vi "Detach Node.vi"(6 "Delete Children?(True)":bool=TRUE, 8 "error in (no error)":errorcluster, 9 "Delete Activate Node(False)":bool, 10 "Node Name":string, 11 "TREE in":refnum<class "MyTreeAPI.lvclass">) -> (0 "error out":errorcluster, 3 "TREE out":refnum<class "MyTreeAPI.lvclass">)   [LabVIEW 2015, in "MyTreeAPI.lvclass"]
uses:
  MyTreeAPI.lvclass
  MyTreeAPI.lvclass/MyTreeAPI.ctl
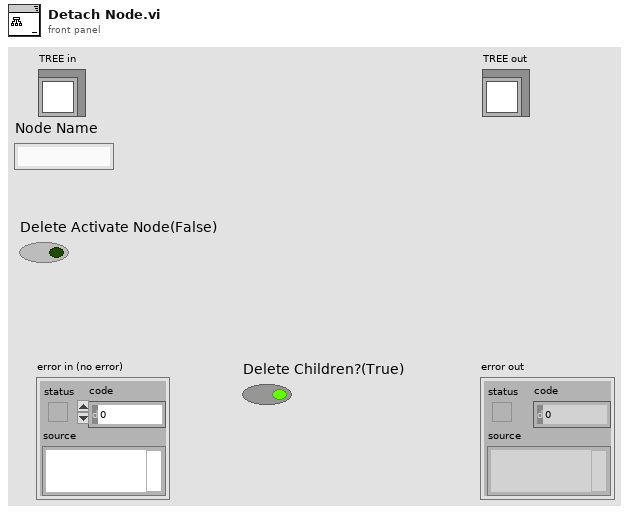
[diagram p1: front panel]
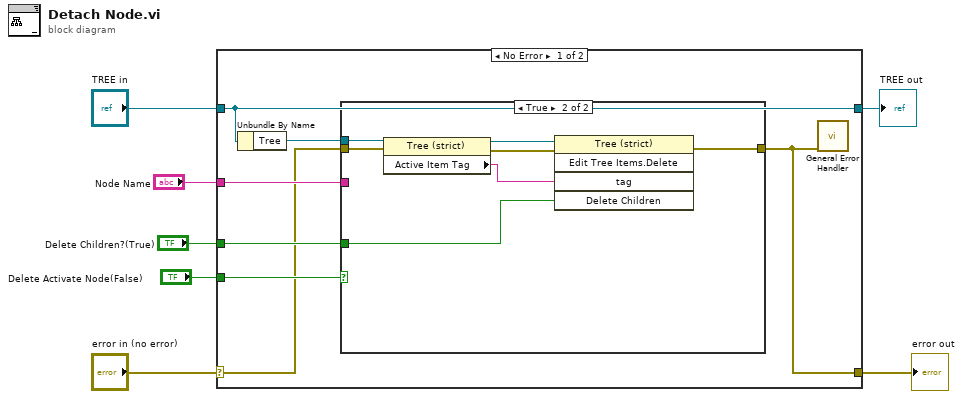
[diagram p0: block diagram]
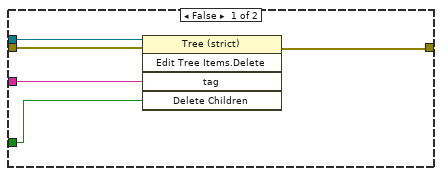
[diagram p2: hidden frame]
diagram:
  n1 = case shown="No Error" "error in (no error)" {
    selector: "error in (no error)" -> [w9 w28]
    tunnel: [w8 w28] -> w6
    tunnel: [w14 w27] -> w4
    tunnel: "TREE in" -> [w14 w27]
    tunnel: "Node Name" -> [w11 _]
    tunnel: "Delete Children?(True)" -> [w10 _]
    tunnel: "Delete Activate Node(False)" -> [w13 _]
    frame No Error {
      n2 = Unbundle By Name(w14) -> ("Tree"=w12:refnum<vi>)
      n3 = case shown="True" w13 {
        tunnel: w12 -> [w19 w26]
        tunnel: w11 -> [w17 _]
        tunnel: w10 -> [w16 w21]
        tunnel: w9 -> [w18 w23]
        tunnel: [w15 w20] -> w8
        frame False {
          n4 = invoke class="Tree (strict)" method="Edit Tree Items.Delete"(reference=w19, error in=w18, "tag"=w17, "Delete Children"=w16) -> (error out=w15:errorcluster)  [unwired: 1 in, 4 out]
        }
        frame True {
          n5 = property class="Tree (strict)"(reference=w26, error in=w23) -> (reference out=w25:refnum<vi>, error out=w24:errorcluster, "Active Item Tag"=w22:string)
          n6 = invoke class="Tree (strict)" method="Edit Tree Items.Delete"(reference=w25, error in=w24, "tag"=w22, "Delete Children"=w21) -> (error out=w20:errorcluster)  [unwired: 1 in, 4 out]
        }
      }
      n7 = call <vilib>:"General Error Handler.vi"("error in (no error)"=w8) -> ()  [unwired: 10 in, 5 out]
    }
    frame Error {
    }
  }
  "error out" <- w6
  "TREE out" <- w4
